vi "4145 Wait on Event  GPIB .vi"(0 "Address":string, 3 "timeout ms":u32=25000, 5 "error in":T1) -> (14 "Stopped":bool, 16 "GPIB error":i16, 19 "error out":errorcluster)   [LabVIEW 2014]
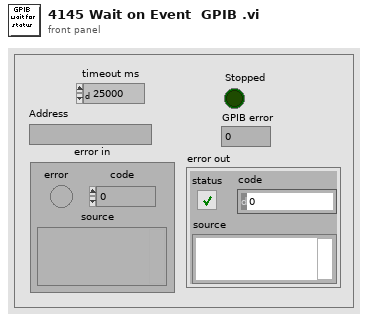
[diagram p1: front panel]
types:
  T1 = cluster{"error":bool, "code":i32, "source":string}
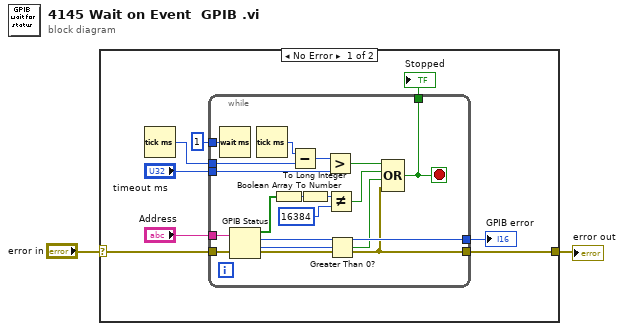
[diagram p0: block diagram]
diagram:
  n1 = case shown="No Error" "error in" {
    selector: "error in" -> [w6 w29]
    tunnel: [w3 w29] -> w1
    frame No Error {
      n2 = Tick Count (ms)() -> (millisecond timer value=w10:u32)
      n3 = while {
        tunnel: w10 -> [w27]
        tunnel: "timeout ms" -> [w25]
        tunnel: [w22] -> w8
        tunnel: "Address" -> [w24]
        tunnel: w6 -> [w15]
        tunnel: [w14] -> w5
        tunnel: u32 1 -> [w12]
        tunnel: [w11] -> w3
        stop <- w22 stop-if-true
        n4 = Wait (ms)(milliseconds to wait=w12) -> ()  [unwired: 1 out]
        n5 = GPIB Status(0:w24, 1:w15) -> (2:w21:bool[], 3:w14:i16, 4:w16:i32, 5:w11:errorcluster)
        n6 = Tick Count (ms)() -> (millisecond timer value=w28:u32)
        n7 = Boolean Array To Number(Boolean array=w21) -> (number=w20:u32)
        n8 = Subtract(x=w28, y=w27) -> (x-y=w26:u32)
        n9 = To Long Integer(number=w20) -> (32bit integer=w18:i32)
        n10 = Greater?(x=w26, y=w25) -> (0:w23:bool)
        n11 = Not Equal?(x=w18, y=16384) -> (x != y?=w17:bool)
        n12 = Greater Than 0?(x=w16) -> (x > 0?=w13:bool)
        n13 = Compound Arithmetic op=OR(w23, w17, w13, w11) -> (w22:bool)
      }
      "Stopped" <- w8
      "GPIB error" <- w5
    }
    frame Error {
    }
  }
  "error out" <- w1
